vi "PicoScope2000ClearFastStreaming.vi"(4 "error in":errorcluster, 7 "handle":i16=1) -> (0 "error out":errorcluster, 3 "handle out":i16)   [LabVIEW 2010]
doc: "Clears ps2000 wrapper Fast Streaming counters and indexs"
uses:
  ps2000Wrap.dll
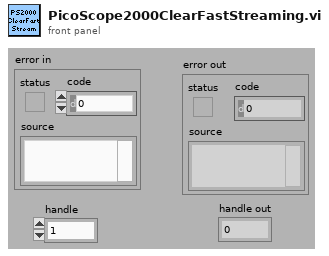
[diagram p1: front panel]
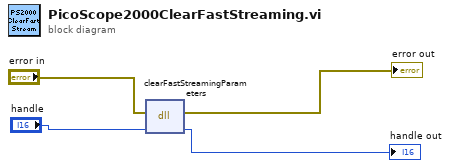
[diagram p0: block diagram]
diagram:
  n1 = dll-call lib="ps2000Wrap.dll" fn="clearFastStreamingParameters"(error in="error in", "handle"="handle") -> (error out=→"error out":errorcluster, "handle"=→"handle out":i16)  [unwired: 3 in, 1 out]
